vi "test - List CSM Modules.vi"(8 "error in (no error)":errorcluster, 11 "TestCase in":refnum<class "testcase-Basic-Function.lvclass">) -> (0 "error out":errorcluster, 3 "TestCase out":refnum<class "testcase-Basic-Function.lvclass">)   [LabVIEW 2017, in "testcase-Basic-Function.lvclass"]
uses:
  testcase-Basic-Function.lvclass
  testcase-Basic-Function.lvclass/testcase-Basic-Function.ctl
  src/user.lib/_NEVSTOP/Communicable State Machine(CSM)/_Support/Typedef/_CSM_List Module Scope.ctl
  42b12831-9811-4844-863c-f1e3d955922c.vi
  <vilib>/addons/_JKI Toolkits/VI Tester/TestCase.llb/TestCase.lvclass
  src/user.lib/_NEVSTOP/Communicable State Machine(CSM)/Communicable State Machine.lvlib
  C:/Program Files (x86)/National Instruments/LabVIEW 2017/vi.lib/addons/_JKI Toolkits/VI Tester/TestCase.llb/TestCase.lvclass
panel:
  out "all":string[](array[string])
  out "Module Names 5":string[](array[string])
  out "normal":string[](array[string])
  out "normal all":string[](array[string])
  out "systemonly all":string[](array[string])
  out "systemonly":string[](array[string])
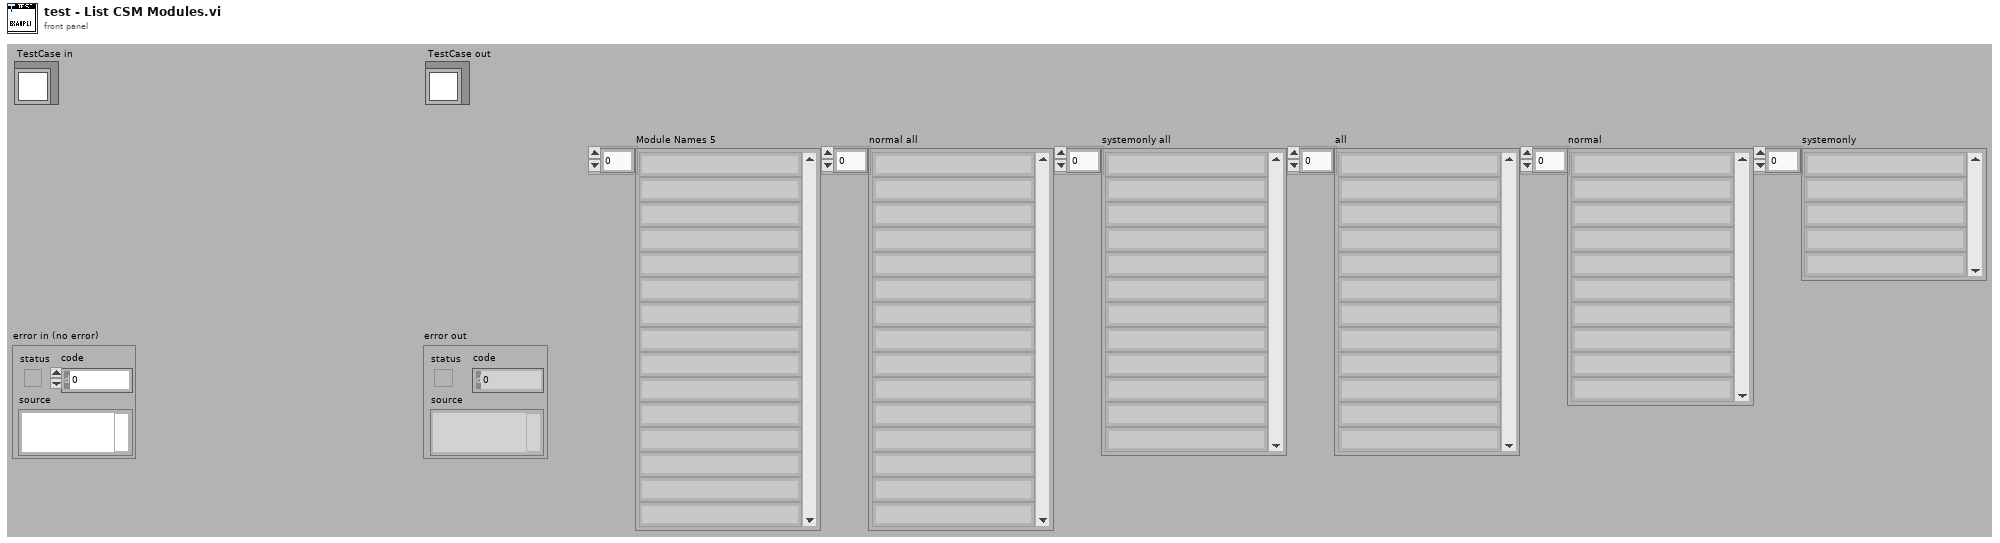
[diagram p1: front panel]
types:
  T1 = typedef "Communicable State Machine.lvlib/_CSM_List Module Scope.ctl" = enum16{"Normal", "System Only", "All"}
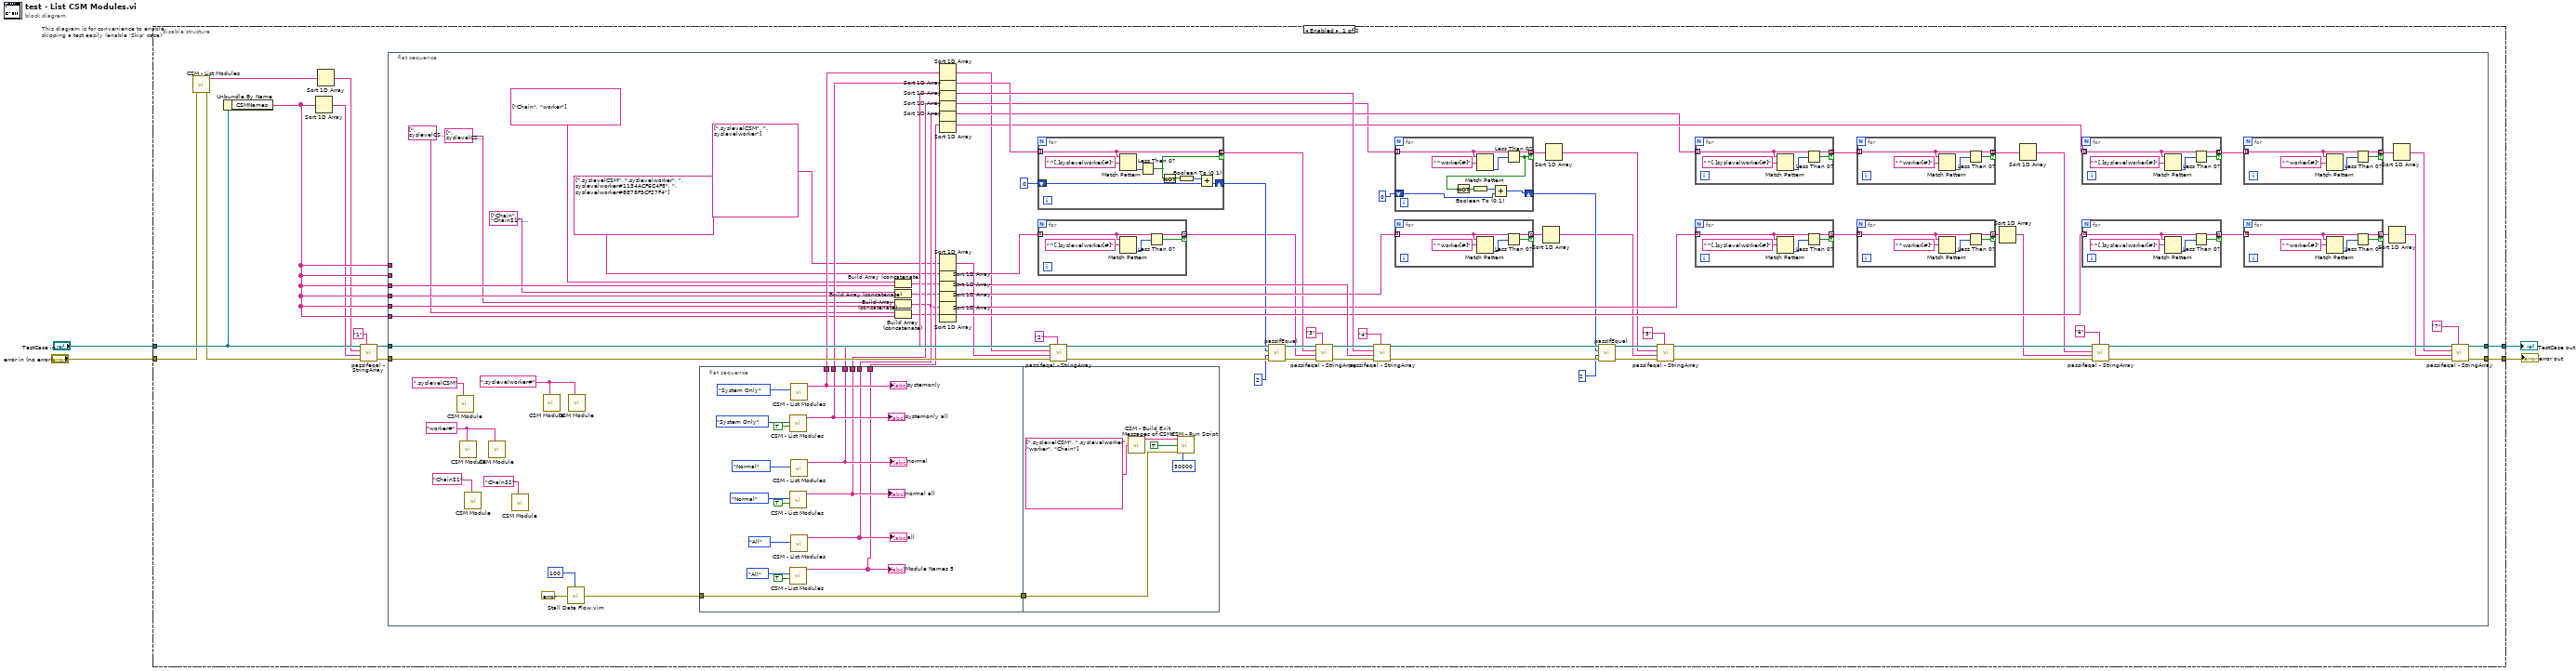
[diagram p0: block diagram]
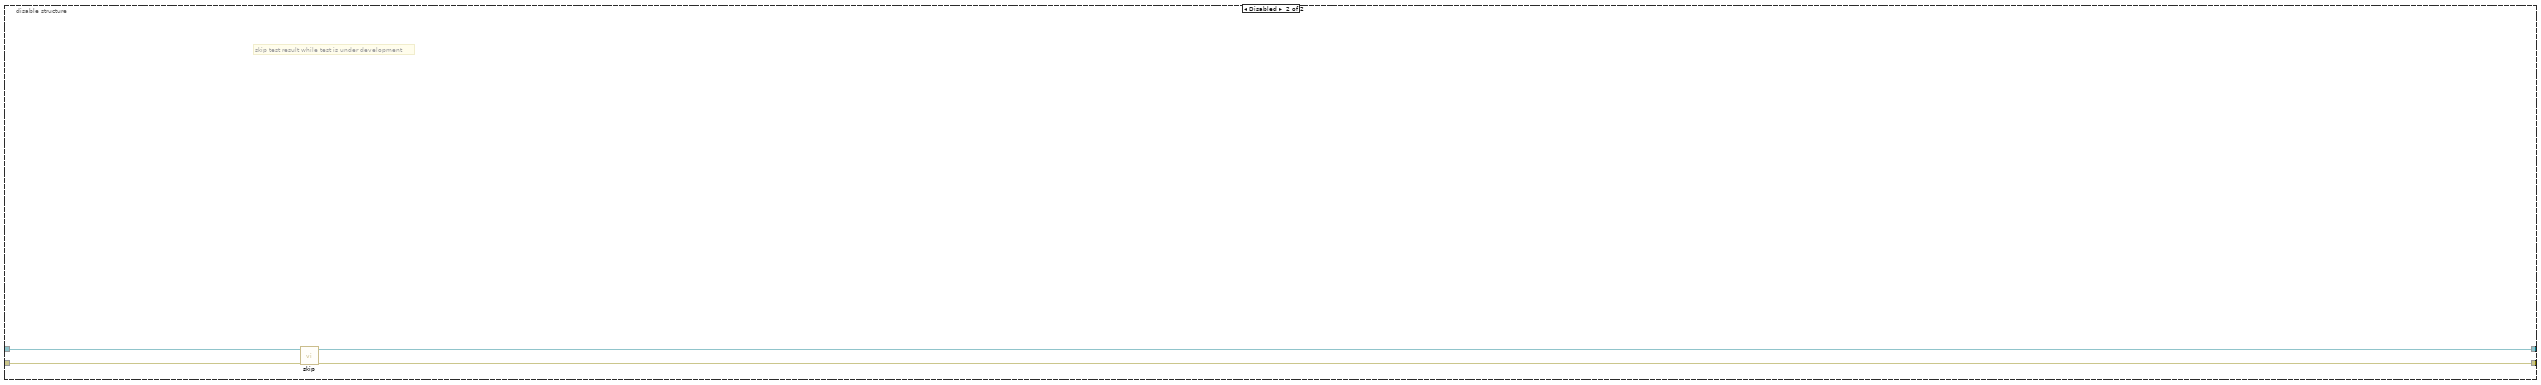
[diagram p2: hidden frame]
diagram:
  n1 = disable-structure "This diagram is for convenience to enable skipping a test easily (enable 'Skip' case)" shown="Enabled" {
    disable-tunnel: "TestCase in" -> [w15 w186]
    disable-tunnel: [w11 w184] -> w1
    disable-tunnel: [w10 w185] -> w3
    disable-tunnel: "error in (no error)" -> [w14 w183]
    frame Enabled {
      n2 = call "CSM - List Modules.vi"("Error In"=w14) -> ("error out"=w13:errorcluster, "Module Names"=w16:string[])  [unwired: 9 in]
      n3 = Unbundle By Name(w15) -> ("CSMNames"=w9:string[])
      n4 = Sort 1D Array(array=w9) -> (sorted array=w6:string[])
      n5 = Sort 1D Array(array=w16) -> (sorted array=w7:string[])
      n6 = call "passifeqal - StringArray.vi"("custom report message (\"\")"="1" ("custom report message (\"\")"), "error in (no error)"=w13, "y"=w6, "x"=w7, "testcase-Basic-Function in"=w15) -> ("error out"=w8:errorcluster, "testcase-Basic-Function out"=w12:refnum<class "testcase-Basic-Function.lvclass">)  [unwired: 4 in]
      n7 = flat-sequence {
        tunnel: [w87] -> w11
        tunnel: [w88] -> w10
        tunnel: w8 -> [w96]
        tunnel: w12 -> [w95]
        tunnel: w9 -> [_]
        tunnel: w9 -> [_]
        tunnel: w9 -> [w80]
        tunnel: w9 -> [w79]
        tunnel: w9 -> [w78]
        tunnel: w9 -> [w77]
        frame #0 {
          w103 = ".syslevelworker#" ("Name (\"\" to Use UUID)")
          w104 = "worker#" ("Name (\"\" to Use UUID)")
          n8 = call "CSM Module.vi"("Name (\"\" to Use UUID)"=".syslevelCSM" ("Name (\"\" to Use UUID)")) -> ()  [unwired: 11 in]
          n9 = call "CSM Module.vi"("Name (\"\" to Use UUID)"=w104) -> ()  [unwired: 11 in]
          n10 = call "CSM Module.vi"("Name (\"\" to Use UUID)"="Chain$1" ("Name (\"\" to Use UUID)")) -> ()  [unwired: 11 in]
          n11 = call "CSM Module.vi"("Name (\"\" to Use UUID)"=w104) -> ()  [unwired: 11 in]
          n12 = call "CSM Module.vi"("Name (\"\" to Use UUID)"="Chain$2" ("Name (\"\" to Use UUID)")) -> ()  [unwired: 11 in]
          n13 = call "CSM Module.vi"("Name (\"\" to Use UUID)"=w103) -> ()  [unwired: 11 in]
          n14 = call "Stall Data Flow.vim"("value in"=errorcluster {"status"=FALSE, "code"=0, "source"=""} ("error in (no error)"), "milliseconds to wait"=u32 100) -> ("value out"=w101:errorcluster)  [unwired: 1 out]
          n15 = call "CSM Module.vi"("Name (\"\" to Use UUID)"=w103) -> ()  [unwired: 11 in]
          n16 = flat-sequence {
            tunnel: w101 -> [w168]
            tunnel: [w168] -> w99
            tunnel: [w167] -> w86
            tunnel: [w166] -> w85
            tunnel: [w165] -> w84
            tunnel: [w164] -> w83
            tunnel: [w163] -> w82
            tunnel: [w162] -> w81
            tunnel: w99 -> [w179]
            frame #0 {
              n17 = call "CSM - List Modules.vi"("With Nodes? (F)"=TRUE ("With Instance(F)"), "Scope (Normal)"=_CSM_List_Module_Scope."System Only" ("Scope(Normal)")) -> ("Module Names"=w166:string[])  [unwired: 8 in, 1 out]
              "systemonly all" <- w166
              n18 = call "CSM - List Modules.vi"("With Nodes? (F)"=TRUE ("With Instance(F)"), "Scope (Normal)"=_CSM_List_Module_Scope."Normal" ("Scope(Normal)")) -> ("Module Names"=w164:string[])  [unwired: 8 in, 1 out]
              "normal all" <- w164
              n19 = call "CSM - List Modules.vi"("With Nodes? (F)"=TRUE ("With Instance(F)"), "Scope (Normal)"=_CSM_List_Module_Scope."All" ("Scope(Normal)")) -> ("Module Names"=w162:string[])  [unwired: 8 in, 1 out]
              "Module Names 5" <- w162
              n20 = call "CSM - List Modules.vi"("Scope (Normal)"=_CSM_List_Module_Scope."System Only" ("Scope(Normal)")) -> ("Module Names"=w167:string[])  [unwired: 9 in, 1 out]
              "systemonly" <- w167
              n21 = call "CSM - List Modules.vi"("Scope (Normal)"=_CSM_List_Module_Scope."Normal" ("Scope(Normal)")) -> ("Module Names"=w165:string[])  [unwired: 9 in, 1 out]
              "normal" <- w165
              n22 = call "CSM - List Modules.vi"("Scope (Normal)"=_CSM_List_Module_Scope."All" ("Scope(Normal)")) -> ("Module Names"=w163:string[])  [unwired: 9 in, 1 out]
              "all" <- w163
            }
            frame #1 {
              n23 = call "CSM - Build Exit Messages of CSMs.vi"("CSMs"=string[] [".syslevelCSM", ".syslevelworker", "worker", "Chain"]) -> ("States"=w182:string)  [unwired: 14 in]
              n24 = call "CSM - Run Script.vi"("CSM Scripts"=w182, "Continue If Error? (F)"=TRUE ("Continue If Error?(F)"), "error in (no error)"=w179, "Response Timeout (-2 Using Global Settings)"=30000) -> ()  [unwired: 9 in, 3 out]
            }
          }
          n25 = Build Array (concatenate)(string[] ["Chain", "worker"] ("normal"), w80) -> (w70:string[])
          n26 = Build Array (concatenate)(string[] ["Chain", "Chain$1", "Chain$2", "worker", "worker#2C89E5CA7D1A", "worker#3ED3210DFA85"] ("normal all"), w79) -> (w69:string[])
          n27 = Build Array (concatenate)(string[] [".syslevelCSM", ".syslevelworker", "Chain", "worker"] ("all"), w78) -> (w68:string[])
          n28 = Build Array (concatenate)(string[] [".syslevelCSM", ".syslevelworker", ".syslevelworker#1134ACF6C4F8", ".syslevelworker#8E78F5CF27F4", "Chain", "Chain$1", "Chain$2", "worker", "worker#2C89E5CA7D1A", "worker#3ED3210DFA85"] ("Module Names 5"), w77) -> (w67:string[])
          n29 = Sort 1D Array(array=w86) -> (sorted array=w24:string[])
          n30 = Sort 1D Array(array=w85) -> (sorted array=w63:string[])
          n31 = Sort 1D Array(array=w84) -> (sorted array=w66:string[])
          n32 = Sort 1D Array(array=w83) -> (sorted array=w50:string[])
          n33 = Sort 1D Array(array=w82) -> (sorted array=w60:string[])
          n34 = Sort 1D Array(array=w81) -> (sorted array=w62:string[])
          n35 = Sort 1D Array(array=string[] [".syslevelCSM", ".syslevelworker"] ("systemonly")) -> (sorted array=w23:string[])
          n36 = Sort 1D Array(array=string[] [".syslevelCSM", ".syslevelworker", ".syslevelworker#1134ACF6C4F8", ".syslevelworker#8E78F5CF27F4"] ("systemonly all")) -> (sorted array=w64:string[])
          n37 = Sort 1D Array(array=w70) -> (sorted array=w65:string[])
          n38 = Sort 1D Array(array=w69) -> (sorted array=w48:string[])
          n39 = Sort 1D Array(array=w68) -> (sorted array=w59:string[])
          n40 = Sort 1D Array(array=w67) -> (sorted array=w61:string[])
          n41 = for {
            tunnel: w63 -> [w160] mode=indexing
            tunnel: [w160] -> w32 mode=indexing if=w156
            shift-right: [w157] -> w41
            shift-left: 0 -> [w158]
            n42 = Match Pattern(string=w160, regular expression="^[.]syslevelworker[#]") -> (offset past match=w159:i32)  [unwired: 1 in, 3 out]
            n43 = Less Than 0?(x=w159) -> (x < 0?=w156:bool)
            n44 = Not(x=w156) -> (.not. x?=w155:bool)
            n45 = Boolean To (0,1)(Boolean=w155) -> (0, 1=w154:i16)
            n46 = Add(x=w154, y=w158) -> (x+y=w157:i32)
          }
          n47 = for {
            tunnel: w64 -> [w152] mode=indexing
            tunnel: [w152] -> w31 mode=indexing if=w150
            n48 = Match Pattern(string=w152, regular expression="^[.]syslevelworker[#]") -> (offset past match=w151:i32)  [unwired: 1 in, 3 out]
            n49 = Less Than 0?(x=w151) -> (x < 0?=w150:bool)
          }
          n50 = call "passifeqal - StringArray.vi"("custom report message (\"\")"="2" ("custom report message (\"\")"), "error in (no error)"=w96, "y"=w23, "x"=w24, "testcase-Basic-Function in"=w95) -> ("error out"=w42:errorcluster, "testcase-Basic-Function out"=w43:refnum<class "testcase-Basic-Function.lvclass">)  [unwired: 4 in]
          n51 = call-dynamic "passIfEqual.vi"("error in (no error)"=w42, "y"=2, "x"=w41, "TestCase in"=w43) -> ("error out"=w45:errorcluster, "TestCase out"=w44:refnum<class "testcase-Basic-Function.lvclass">)  [unwired: 6 in]
          n52 = call "passifeqal - StringArray.vi"("custom report message (\"\")"="3" ("custom report message (\"\")"), "error in (no error)"=w45, "y"=w31, "x"=w32, "testcase-Basic-Function in"=w44) -> ("error out"=w93:errorcluster, "testcase-Basic-Function out"=w94:refnum<class "testcase-Basic-Function.lvclass">)  [unwired: 4 in]
          n53 = call "passifeqal - StringArray.vi"("custom report message (\"\")"="4" ("custom report message (\"\")"), "error in (no error)"=w93, "y"=w65, "x"=w66, "testcase-Basic-Function in"=w94) -> ("error out"=w35:errorcluster, "testcase-Basic-Function out"=w36:refnum<class "testcase-Basic-Function.lvclass">)  [unwired: 4 in]
          n54 = for {
            tunnel: w50 -> [w116] mode=indexing
            tunnel: [w116] -> w49 mode=indexing if=w112
            shift-right: [w110] -> w33
            shift-left: 0 -> [w111]
            n55 = Match Pattern(string=w116, regular expression="^worker[#]") -> (offset past match=w115:i32)  [unwired: 1 in, 3 out]
            n56 = Less Than 0?(x=w115) -> (x < 0?=w112:bool)
            n57 = Not(x=w112) -> (.not. x?=w114:bool)
            n58 = Boolean To (0,1)(Boolean=w114) -> (0, 1=w113:i16)
            n59 = Add(x=w113, y=w111) -> (x+y=w110:i32)
          }
          n60 = for {
            tunnel: w48 -> [w108] mode=indexing
            tunnel: [w108] -> w47 mode=indexing if=w106
            n61 = Match Pattern(string=w108, regular expression="^worker[#]") -> (offset past match=w107:i32)  [unwired: 1 in, 3 out]
            n62 = Less Than 0?(x=w107) -> (x < 0?=w106:bool)
          }
          n63 = Sort 1D Array(array=w47) -> (sorted array=w29:string[])
          n64 = Sort 1D Array(array=w49) -> (sorted array=w30:string[])
          n65 = call-dynamic "passIfEqual.vi"("error in (no error)"=w35, "y"=2, "x"=w33, "TestCase in"=w36) -> ("error out"=w37:errorcluster, "TestCase out"=w38:refnum<class "testcase-Basic-Function.lvclass">)  [unwired: 6 in]
          n66 = call "passifeqal - StringArray.vi"("custom report message (\"\")"="5" ("custom report message (\"\")"), "error in (no error)"=w37, "y"=w29, "x"=w30, "testcase-Basic-Function in"=w38) -> ("error out"=w91:errorcluster, "testcase-Basic-Function out"=w92:refnum<class "testcase-Basic-Function.lvclass">)  [unwired: 4 in]
          n67 = for {
            tunnel: w60 -> [w140] mode=indexing
            tunnel: [w140] -> w58 mode=indexing if=w138
            n68 = Match Pattern(string=w140, regular expression="^[.]syslevelworker[#]") -> (offset past match=w139:i32)  [unwired: 1 in, 3 out]
            n69 = Less Than 0?(x=w139) -> (x < 0?=w138:bool)
          }
          n70 = for {
            tunnel: w59 -> [w136] mode=indexing
            tunnel: [w136] -> w57 mode=indexing if=w134
            n71 = Match Pattern(string=w136, regular expression="^[.]syslevelworker[#]") -> (offset past match=w135:i32)  [unwired: 1 in, 3 out]
            n72 = Less Than 0?(x=w135) -> (x < 0?=w134:bool)
          }
          n73 = for {
            tunnel: w58 -> [w124] mode=indexing
            tunnel: [w124] -> w55 mode=indexing if=w122
            n74 = Match Pattern(string=w124, regular expression="^worker[#]") -> (offset past match=w123:i32)  [unwired: 1 in, 3 out]
            n75 = Less Than 0?(x=w123) -> (x < 0?=w122:bool)
          }
          n76 = for {
            tunnel: w57 -> [w120] mode=indexing
            tunnel: [w120] -> w56 mode=indexing if=w118
            n77 = Match Pattern(string=w120, regular expression="^worker[#]") -> (offset past match=w119:i32)  [unwired: 1 in, 3 out]
            n78 = Less Than 0?(x=w119) -> (x < 0?=w118:bool)
          }
          n79 = Sort 1D Array(array=w56) -> (sorted array=w27:string[])
          n80 = Sort 1D Array(array=w55) -> (sorted array=w28:string[])
          n81 = for {
            tunnel: w62 -> [w148] mode=indexing
            tunnel: [w148] -> w54 mode=indexing if=w146
            n82 = Match Pattern(string=w148, regular expression="^[.]syslevelworker[#]") -> (offset past match=w147:i32)  [unwired: 1 in, 3 out]
            n83 = Less Than 0?(x=w147) -> (x < 0?=w146:bool)
          }
          n84 = for {
            tunnel: w61 -> [w144] mode=indexing
            tunnel: [w144] -> w53 mode=indexing if=w142
            n85 = Match Pattern(string=w144, regular expression="^[.]syslevelworker[#]") -> (offset past match=w143:i32)  [unwired: 1 in, 3 out]
            n86 = Less Than 0?(x=w143) -> (x < 0?=w142:bool)
          }
          n87 = call "passifeqal - StringArray.vi"("custom report message (\"\")"="6" ("custom report message (\"\")"), "error in (no error)"=w91, "y"=w27, "x"=w28, "testcase-Basic-Function in"=w92) -> ("error out"=w89:errorcluster, "testcase-Basic-Function out"=w90:refnum<class "testcase-Basic-Function.lvclass">)  [unwired: 4 in]
          n88 = for {
            tunnel: w54 -> [w132] mode=indexing
            tunnel: [w132] -> w51 mode=indexing if=w130
            n89 = Match Pattern(string=w132, regular expression="^worker[#]") -> (offset past match=w131:i32)  [unwired: 1 in, 3 out]
            n90 = Less Than 0?(x=w131) -> (x < 0?=w130:bool)
          }
          n91 = for {
            tunnel: w53 -> [w128] mode=indexing
            tunnel: [w128] -> w52 mode=indexing if=w126
            n92 = Match Pattern(string=w128, regular expression="^worker[#]") -> (offset past match=w127:i32)  [unwired: 1 in, 3 out]
            n93 = Less Than 0?(x=w127) -> (x < 0?=w126:bool)
          }
          n94 = Sort 1D Array(array=w52) -> (sorted array=w25:string[])
          n95 = Sort 1D Array(array=w51) -> (sorted array=w26:string[])
          n96 = call "passifeqal - StringArray.vi"("custom report message (\"\")"="7" ("custom report message (\"\")"), "error in (no error)"=w89, "y"=w25, "x"=w26, "testcase-Basic-Function in"=w90) -> ("error out"=w88:errorcluster, "testcase-Basic-Function out"=w87:refnum<class "testcase-Basic-Function.lvclass">)  [unwired: 4 in]
        }
      }
    }
    frame Disabled {
      # "skip test result while test is under development"
      n97 = call <vilib>:"skip.vi"("error in (no error)"=w183, "TestCase in"=w186) -> ("error out"=w185:errorcluster, "TestCase out"=w184:refnum<class "testcase-Basic-Function.lvclass">)  [unwired: 8 in]
    }
  }
  "error out" <- w3
  "TestCase out" <- w1
